vi "Pos_iniciales.vi"() -> ()   [LabVIEW 2020]
panel:
  in  "Pos_Iniciales":T1
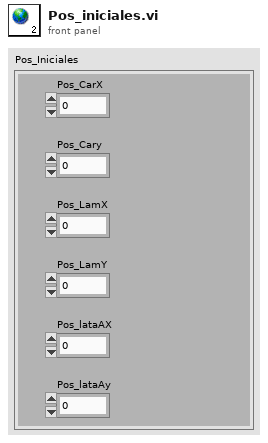
[diagram p1: front panel]
types:
  T1 = cluster{"Pos_CarX":dbl, "Pos_Cary":dbl, "Pos_LamX":dbl, "Pos_LamY":dbl, "Pos_lataAX":dbl, "Pos_lataAy":dbl}
diagram:
